vi "Tetris_GameLogicLoop.vi"   [LabVIEW 2018]
uses:
  TypDefs/State_Enum.ctl
  TypDefs/Joystick_Enum.ctl
  <vilib>/rvi/Emulation/niFpgaGetClockAttributes.vi
  <vilib>/rvi/Emulation/niFpgaSctlEmulationGetInTimedLoop.vi
  <vilib>/rvi/Emulation/niFpgaEmulationReportErrorSimple.vi
  Control_GameOverGlobal.vi
  <vilib>/rvi/Emulation/niFpgaProcessEmulError.vi
  <vilib>/rvi/Emulation/niFpgaCriticalErrorInLSC.vi
types:
  T1 = typedef "State_Enum.ctl" = enum8{"Wait for Start", "Initialize Game", "Copy Game- to DrawPlayfield", "Place Tetro on GamePlayfield", "Place Tetro on DrawPlayfield", "Create Tetromino", "Check if GameOver", "Freeze Game", "Check DropTimer", "Check Joystick", "Detect Collision", "Move Tetromino", "Clear Full Lines", "Update Score", "Check for Perfect Clear"}
  T2 = typedef "Joystick_Enum.ctl" = enum8{"Button", "Left", "Right", "Up", "Down", "None"}
  T3 = cluster{"State":T1, "Joystick":T2, "Origin":i16, "Tetromino":u8, "LinesCleared":u8, "Score":i16, "Timer.t0":u16, "CreateNewTetro":bool}[]
  T4 = cluster{"State":T1, "Joystick":T2, "Origin":i16, "Tetromino":u8, "LinesCleared":u8, "Score":i16, "Timer.t0":u16, "CreateNewTetro":bool}
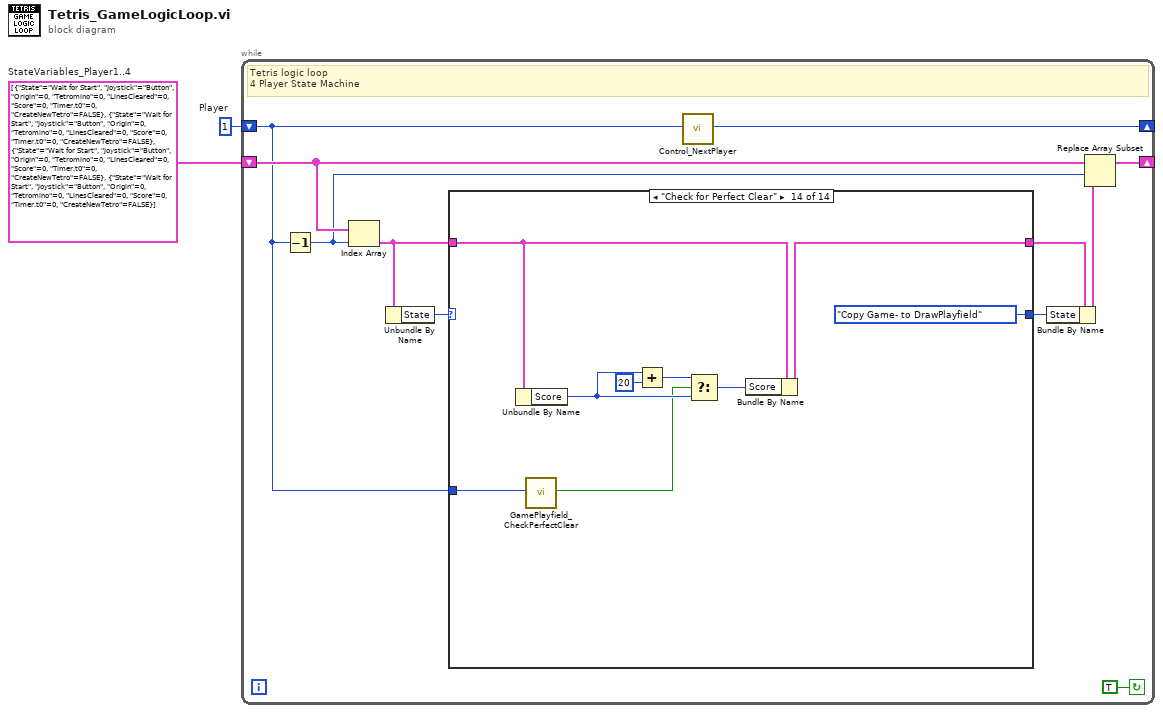
[diagram p0: block diagram]
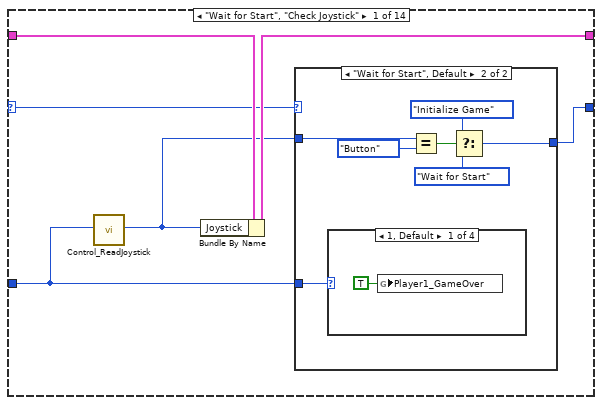
[diagram p2: hidden frame]
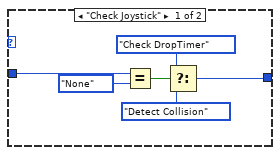
[diagram p3: hidden frame]
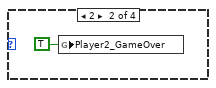
[diagram p4: hidden frame]
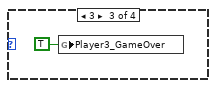
[diagram p5: hidden frame]
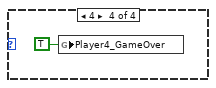
[diagram p6: hidden frame]
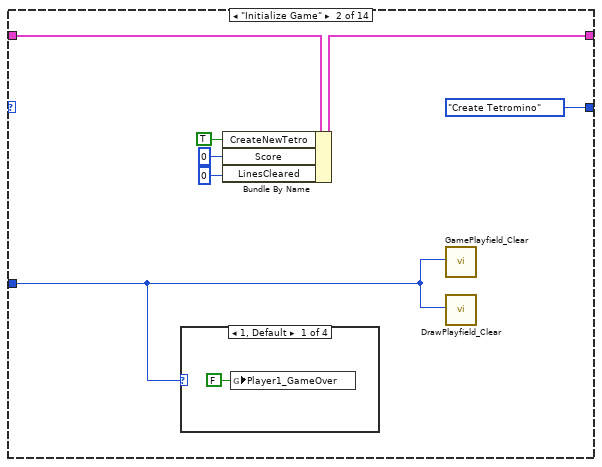
[diagram p7: hidden frame]
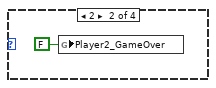
[diagram p8: hidden frame]
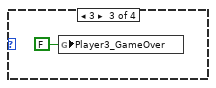
[diagram p9: hidden frame]
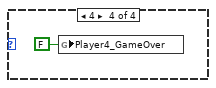
[diagram p10: hidden frame]
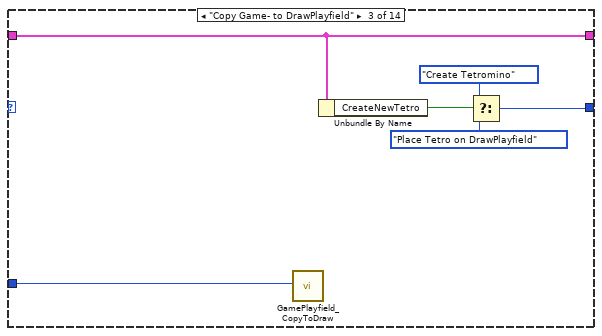
[diagram p11: hidden frame]
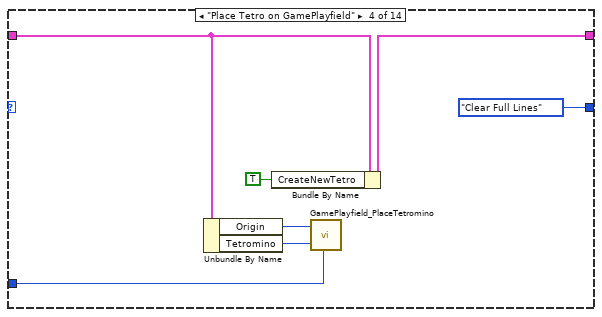
[diagram p12: hidden frame]
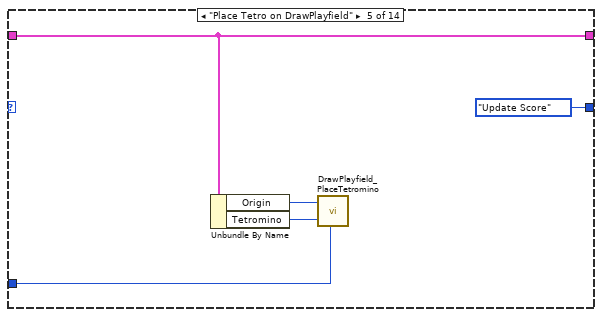
[diagram p13: hidden frame]
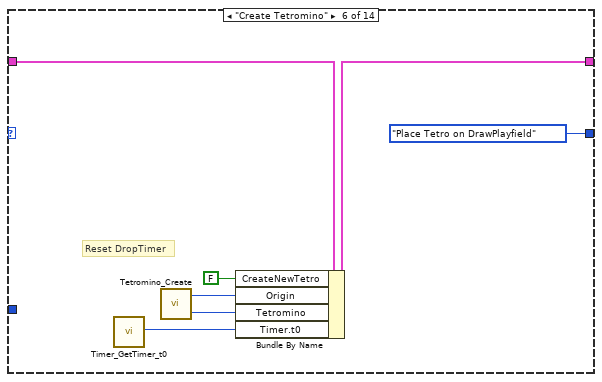
[diagram p14: hidden frame]
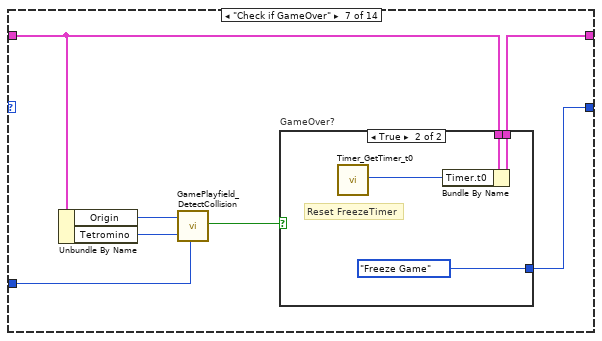
[diagram p15: hidden frame]
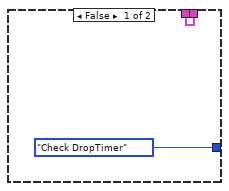
[diagram p16: hidden frame]
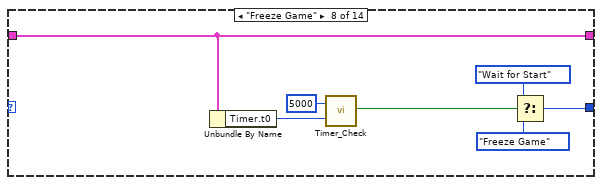
[diagram p17: hidden frame]
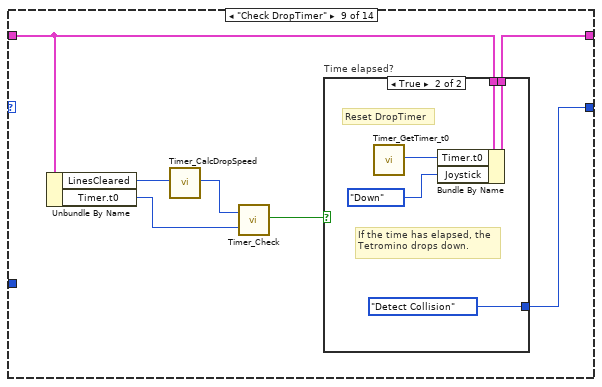
[diagram p18: hidden frame]
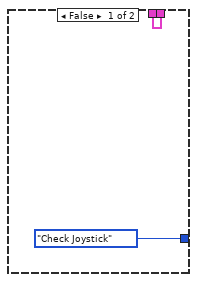
[diagram p19: hidden frame]
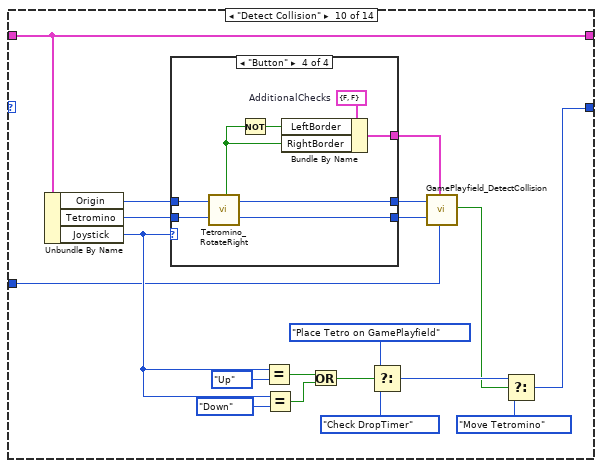
[diagram p20: hidden frame]
diagram:
  w1 = u8 1  # Player
  w2 = T3 [{"State"=enum."Wait for Start", "Joystick"=enum."Button", "Origin"=0, "Tetromino"=0, "LinesCleared"=0, "Score"=0, "Timer.t0"=0, "CreateNewTetro"=FALSE}, {"State"=enum."Wait for Start", "Joystick"=enum."Button", "Origin"=0, "Tetromino"=0, "LinesCleared"=0, "Score"=0, "Timer.t0"=0, "CreateNewTetro"=FALSE}, {"State"=enum."Wait for Start", "Joystick"=enum."Button", "Origin"=0, "Tetromino"=0, "LinesCleared"=0, "Score"=0, "Timer.t0"=0, "CreateNewTetro"=FALSE}, {"State"=enum."Wait for Start", "Joystick"=enum."Button", "Origin"=0, "Tetromino"=0, "LinesCleared"=0, "Score"=0, "Timer.t0"=0, "CreateNewTetro"=FALSE}]  # StateVariables_Player1..4
  n1 = while {
    shift-right: [w7] -> _
    shift-left: w2 -> [w8]
    shift-right: [w3] -> _
    shift-left: w1 -> [w4]
    stop <- TRUE continue-if-true
    # "Tetris logic loop\n4 Player State Machine"
    n2 = Decrement(x=w4) -> (x-1=w5:u8)
    n3 = Index Array(array=w8, index=w5) -> (element=w9:T4)
    n4 = Unbundle By Name(w9) -> ("State"=w12:T1)
    n5 = case shown="\"Check for Perfect Clear\"" w12 {
      selector: w12 -> [w16 _ _ _ _ _ _ _ _ _ _ _ _ _]
      tunnel: [w17 w42 w51 w59 w62 w68 w75 w92 w99 w115 w155 w180 w188 w196] -> w11
      tunnel: w9 -> [w19 w43 w51 w60 w62 w72 w76 w92 w98 w115 w154 w181 w188 w197]
      tunnel: [w18 State_Enum."Create Tetromino" ("State") w53 State_Enum."Clear Full Lines" ("State") State_Enum."Update Score" ("State") State_Enum."Place Tetro on DrawPlayfield" ("f") w74 w89 w93 w116 w157 State_Enum."Check for Perfect Clear" ("f") State_Enum."Check if GameOver" ("f") State_Enum."Copy Game- to DrawPlayfield" ("f")] -> w10
      tunnel: w4 -> [w14 w40 w52 w55 w63 _ w73 _ _ w108 w146 w178 w189 w198]
      frame "Wait for Start", "Check Joystick" {
        n6 = call "Control_ReadJoystick.vi"("Player"=w14) -> ("Joystick"=w15:T2)  [unwired: 18 in]
        n7 = Bundle By Name(cluster=w19, "Joystick"=w15) -> (w17:T4)
        n8 = case shown="\"Wait for Start\", Default" w16 {
          tunnel: [w23 w31] -> w18
          tunnel: w15 -> [w21 w30]
          tunnel: w14 -> [_ w26]
          frame "Check Joystick" {
            n9 = Equal?(x=w21, y=Joystick_Enum."None") -> (x = y?=w22:bool)
            n10 = Select(t=State_Enum."Check DropTimer" ("f"), s=w22, f=State_Enum."Detect Collision") -> (s? t:f=w23:T1)
          }
          frame "Wait for Start", Default {
            n11 = case shown="1, Default" w26 {
              frame 1, Default {
                n12 = global write "Control_GameOverGlobal.vi" "Player1_GameOver"(TRUE ("Player1_GameOver")) -> ()
              }
              frame 2 {
                n13 = global write "Control_GameOverGlobal.vi" "Player2_GameOver"(TRUE ("Player1_GameOver")) -> ()
              }
              frame 3 {
                n14 = global write "Control_GameOverGlobal.vi" "Player3_GameOver"(TRUE ("Player1_GameOver")) -> ()
              }
              frame 4 {
                n15 = global write "Control_GameOverGlobal.vi" "Player4_GameOver"(TRUE ("Player1_GameOver")) -> ()
              }
            }
            n16 = Equal?(x=w30, y=Joystick_Enum."Button") -> (x = y?=w27:bool)
            n17 = Select(t=State_Enum."Initialize Game" ("State"), s=w27, f=State_Enum."Wait for Start") -> (s? t:f=w31:T1)
          }
        }
      }
      frame "Initialize Game" {
        n18 = case shown="1, Default" w40 {
          frame 1, Default {
            n19 = global write "Control_GameOverGlobal.vi" "Player1_GameOver"(FALSE ("Player1_GameOver")) -> ()
          }
          frame 2 {
            n20 = global write "Control_GameOverGlobal.vi" "Player2_GameOver"(FALSE ("Player1_GameOver")) -> ()
          }
          frame 3 {
            n21 = global write "Control_GameOverGlobal.vi" "Player3_GameOver"(FALSE ("Player1_GameOver")) -> ()
          }
          frame 4 {
            n22 = global write "Control_GameOverGlobal.vi" "Player4_GameOver"(FALSE ("Player1_GameOver")) -> ()
          }
        }
        n23 = Bundle By Name(cluster=w43, "CreateNewTetro"=TRUE, "Score"=i16 0, "LinesCleared"=u8 0) -> (w42:T4)
        n24 = call "GamePlayfield_Clear.vi"("Player"=w40) -> ()  [unwired: 19 in]
        n25 = call "DrawPlayfield_Clear.vi"("Player"=w40) -> ()  [unwired: 19 in]
      }
      frame "Copy Game- to DrawPlayfield" {
        n26 = call "GamePlayfield_CopyToDraw.vi"("Player"=w52) -> ()  [unwired: 19 in]
        n27 = Unbundle By Name(w51) -> ("CreateNewTetro"=w50:bool)
        n28 = Select(t=State_Enum."Create Tetromino", s=w50, f=State_Enum."Place Tetro on DrawPlayfield") -> (s? t:f=w53:T1)
      }
      frame "Place Tetro on GamePlayfield" {
        n29 = Unbundle By Name(w60) -> ("Origin"=w57:i16, "Tetromino"=w56:u8)
        n30 = Bundle By Name(cluster=w60, "CreateNewTetro"=TRUE ("CreateTetromino")) -> (w59:T4)
        n31 = call "GamePlayfield_PlaceTetromino.vi"("Origin"=w57, "Tetromino"=w56, "Player"=w55) -> ()  [unwired: 17 in]
      }
      frame "Place Tetro on DrawPlayfield" {
        n32 = Unbundle By Name(w62) -> ("Origin"=w65:i16, "Tetromino"=w64:u8)
        n33 = call "DrawPlayfield_PlaceTetromino.vi"("Origin"=w65, "Tetromino"=w64, "Player"=w63) -> ()  [unwired: 17 in]
      }
      frame "Create Tetromino" {
        # "Reset DropTimer"
        n34 = call "Timer_GetTimer_t0.vi"() -> ("Timer.t0"=w66:u16)  [unwired: 19 in]
        n35 = call "Tetromino_Create.vi"() -> ("Origin"=w70:i16, "Tetromino"=w69:u8)  [unwired: 18 in]
        n36 = Bundle By Name(cluster=w72, "CreateNewTetro"=FALSE, "Origin"=w70, "Tetromino"=w69, "Timer.t0"=w66) -> (w68:T4)
      }
      frame "Check if GameOver" {
        n37 = Unbundle By Name(w76) -> ("Origin"=w79:i16, "Tetromino"=w78:u8)
        n38 = call "GamePlayfield_DetectCollision.vi"("Origin"=w79, "Tetromino"=w78, "Player"=w73) -> ("Collision"=w77:bool)  [unwired: 16 in]
        n39 = case "GameOver?" shown="True" w77 {
          tunnel: w76 -> [w81 w85]
          tunnel: [w81 w84] -> w75
          tunnel: [State_Enum."Check DropTimer" ("f") State_Enum."Freeze Game" ("f")] -> w74
          frame False {
          }
          frame True {
            # "Reset FreezeTimer"
            n40 = call "Timer_GetTimer_t0.vi"() -> ("Timer.t0"=w83:u16)  [unwired: 19 in]
            n41 = Bundle By Name(cluster=w85, "Timer.t0"=w83) -> (w84:T4)
          }
        }
      }
      frame "Freeze Game" {
        n42 = Unbundle By Name(w92) -> ("Timer.t0"=w88:u16)
        n43 = call "Timer_Check.vi"("TimeLimit(ms)"=u16 5000, "Timer.t0"=w88) -> ("TimeElapsed"=w86:bool)  [unwired: 17 in]
        n44 = Select(t=State_Enum."Wait for Start" ("f"), s=w86, f=State_Enum."Freeze Game") -> (s? t:f=w89:T1)
      }
      frame "Check DropTimer" {
        n45 = Unbundle By Name(w98) -> ("LinesCleared"=w97:u8, "Timer.t0"=w95:u16)
        n46 = call "Timer_CalcDropSpeed.vi"("LinesCleared"=w97) -> ("DropSpeed(ms)"=w96:u16)  [unwired: 18 in]
        n47 = call "Timer_Check.vi"("TimeLimit(ms)"=w96, "Timer.t0"=w95) -> ("TimeElapsed"=w94:bool)  [unwired: 17 in]
        n48 = case "Time elapsed?" shown="True" w94 {
          tunnel: [w100 w106] -> w99
          tunnel: w98 -> [w100 w105]
          tunnel: [State_Enum."Check Joystick" ("f") State_Enum."Detect Collision" ("f")] -> w93
          frame False {
          }
          frame True {
            # "If the time has elapsed, the\nTetromino drops down."
            # "Reset DropTimer"
            n49 = call "Timer_GetTimer_t0.vi"() -> ("Timer.t0"=w103:u16)  [unwired: 19 in]
            n50 = Bundle By Name(cluster=w105, "Timer.t0"=w103, "Joystick"=Joystick_Enum."Down") -> (w106:T4)
          }
        }
      }
      frame "Detect Collision" {
        n51 = Unbundle By Name(w115) -> ("Origin"=w112:i16, "Tetromino"=w110:u8, "Joystick"=w113:T2)
        n52 = case shown="\"Button\"" w113 {
          tunnel: w112 -> [w129 w133 w137 w142]
          tunnel: [w128 w132 w136 w138] -> w107
          tunnel: [w127 w131 w135 w141] -> w111
          tunnel: w110 -> [w126 w130 w134 w144]
          tunnel: [w126 w130 w134 w143] -> w109
          frame "Left", Default {
            w127 = cluster{"LeftBorder":bool, "RightBorder":bool} {"LeftBorder"=TRUE, "RightBorder"=FALSE}  # AdditionalChecks
            n53 = call "Tetromino_MoveLeft.vi"("Origin"=w129) -> ("NewOrigin"=w128:i16)  [unwired: 18 in]
          }
          frame "Right" {
            w131 = cluster{"LeftBorder":bool, "RightBorder":bool} {"LeftBorder"=FALSE, "RightBorder"=TRUE}  # AdditionalChecks
            n54 = call "Tetromino_MoveRight.vi"("Origin"=w133) -> ("NewOrigin"=w132:i16)  [unwired: 18 in]
          }
          frame "Up", "Down" {
            w135 = cluster{"LeftBorder":bool, "RightBorder":bool} {"LeftBorder"=FALSE, "RightBorder"=FALSE}  # AdditionalChecks
            n55 = call "Tetromino_MoveDown.vi"("Origin"=w137) -> ("NewOrigin"=w136:i16)  [unwired: 18 in]
          }
          frame "Button" {
            w145 = cluster{"LeftBorder":bool, "RightBorder":bool} {"LeftBorder"=FALSE, "RightBorder"=FALSE}  # AdditionalChecks
            n56 = call "Tetromino_RotateRight.vi"("Origin IN"=w142, "Tetromino"=w144) -> ("CheckBorder\nT = RightSide\nF = LeftSide"=w139:bool, "Origin OUT"=w138:i16, "RotatedTetromino"=w143:u8)  [unwired: 15 in]
            n57 = Not(x=w139) -> (.not. x?=w140:bool)
            n58 = Bundle By Name(cluster=w145, "LeftBorder"=w140, "RightBorder"=w139) -> (w141:cluster{"LeftBorder":bool, "RightBorder":bool})
          }
        }
        n59 = Equal?(x=w113, y=Joystick_Enum."Up") -> (x = y?=w123:bool)
        n60 = Equal?(x=w113, y=Joystick_Enum."Down") -> (x = y?=w122:bool)
        n61 = Or(x=w123, y=w122) -> (x .or. y?=w121:bool)
        n62 = Select(t=State_Enum."Place Tetro on GamePlayfield" ("f"), s=w121, f=State_Enum."Check DropTimer") -> (s? t:f=w119:T1)
        n63 = call "GamePlayfield_DetectCollision.vi"("Origin"=w107, "Tetromino"=w109, "AdditionalChecks"=w111, "Player"=w108) -> ("Collision"=w114:bool)  [unwired: 15 in]
        n64 = Select(t=w119, s=w114, f=State_Enum."Move Tetromino") -> (s? t:f=w116:T1)
      }
      frame "Move Tetromino" {
        n65 = Unbundle By Name(w154) -> ("Joystick"=w151:T2, "Origin"=w150:i16, "Tetromino"=w149:u8)
        n66 = call "UserLED_Toggle.vi"("Player"=w146) -> ()  [unwired: 19 in]
        n67 = case shown="\"Left\", Default" w151 {
          tunnel: w150 -> [w161 w164 w167 w169]
          tunnel: w149 -> [w159 w162 w165 w171]
          tunnel: [w160 w163 w166 w168] -> w148
          tunnel: [w159 w162 w165 w170] -> w147
          frame "Left", Default {
            n68 = call "Tetromino_MoveLeft.vi"("Origin"=w161) -> ("NewOrigin"=w160:i16)  [unwired: 18 in]
          }
          frame "Right" {
            n69 = call "Tetromino_MoveRight.vi"("Origin"=w164) -> ("NewOrigin"=w163:i16)  [unwired: 18 in]
          }
          frame "Up", "Down" {
            n70 = call "Tetromino_MoveDown.vi"("Origin"=w167) -> ("NewOrigin"=w166:i16)  [unwired: 18 in]
          }
          frame "Button" {
            n71 = call "Tetromino_RotateRight.vi"("Origin IN"=w169, "Tetromino"=w171) -> ("Origin OUT"=w168:i16, "RotatedTetromino"=w170:u8)  [unwired: 15 in, 1 out]
          }
        }
        n72 = Bundle By Name(cluster=w154, "Origin"=w148, "Tetromino"=w147) -> (w155:T4)
        n73 = Equal?(x=w151, y=Joystick_Enum."Up") -> (x = y?=w153:bool)
        n74 = Select(t=State_Enum."Detect Collision" ("f"), s=w153, f=State_Enum."Copy Game- to DrawPlayfield") -> (s? t:f=w157:T1)
      }
      frame "Clear Full Lines" {
        n75 = Unbundle By Name(w181) -> ("LinesCleared"=w179:u8, "Score"=w174:i16)
        n76 = call "GamePlayfield_LineClear.vi"("Player"=w178) -> ("LinesCleared"=w173:u8)  [unwired: 18 in]
        n77 = case shown="0, Default" w173 {
          tunnel: [i16 0 i16 1 i16 3 i16 5 i16 8] -> w172
          frame 0, Default {
          }
          frame 1 {
          }
          frame 2 {
          }
          frame 3 {
          }
          frame 4 {
          }
        }
        n78 = Add(x=w174, y=w172) -> (x+y=w175:i16)
        n79 = Add(x=w179, y=w173) -> (x+y=w177:u8)
        n80 = Bundle By Name(cluster=w181, "LinesCleared"=w177, "Score"=w175) -> (w180:T4)
      }
      frame "Update Score" {
        n81 = Unbundle By Name(w188) -> ("Score"=w187:i16)
        n82 = call "Score_Update.vi"("Score"=w187, "Player"=w189) -> ()  [unwired: 18 in]
      }
      frame "Check for Perfect Clear" {
        n83 = Unbundle By Name(w197) -> ("Score"=w193:i16)
        n84 = call "GamePlayfield_CheckPerfectClear.vi"("Player"=w198) -> ("PerfectClear"=w191:bool)  [unwired: 18 in]
        n85 = Add(x=w193, y=i16 20) -> (x+y=w194:i16)
        n86 = Select(t=w194, s=w191, f=w193) -> (s? t:f=w195:i16)
        n87 = Bundle By Name(cluster=w197, "Score"=w195) -> (w196:T4)
      }
    }
    n88 = call "Control_NextPlayer.vi"("Player"=w4) -> ("NextPlayer"=w3:u8)  [unwired: 18 in]
    n89 = Bundle By Name(cluster=w11, "State"=w10) -> (w6:T4)
    n90 = Replace Array Subset(array=w8, new element=w6, index=w5) -> (w7:T3)
  }
